vi "Client(UtilityMode).vi"() -> ()   [LabVIEW 2013, in "OPC UA Demo.lvlib"]
doc: "Demonstrates the use of the <B>OPC UA Client VIs</B> to programmatically create an OPC UA client and connects the OPC UA client to an OPC UA server."
uses:
  OPC UA Demo.lvlib
  <vilib>/OPCUA/client/Write Int32.vi
  <vilib>/OPCUA/NI OPC UA Client.lvlib
  OPCUA(Utility)/Client/OCPUA Client(UtilityMode).lvlib
panel:
  in  "Device.Node.Set Point":i32=1000
  out "error out":errorcluster
  out "Waveform Chart":i32(graph)
  in  "stop":bool
  # "Overview: Demonstrates the use of the OPC UA Client VIs to programmatically create an OPC UA client and connects the OPC UA client to an OPC UA server.\nRequirements: \n1. LabVIEW Datalogging and Supervisory Control Module or LabVIEW Real-Time Module\n2. (Real-Time Module) RT target\nInstructions:\nRun the VI."
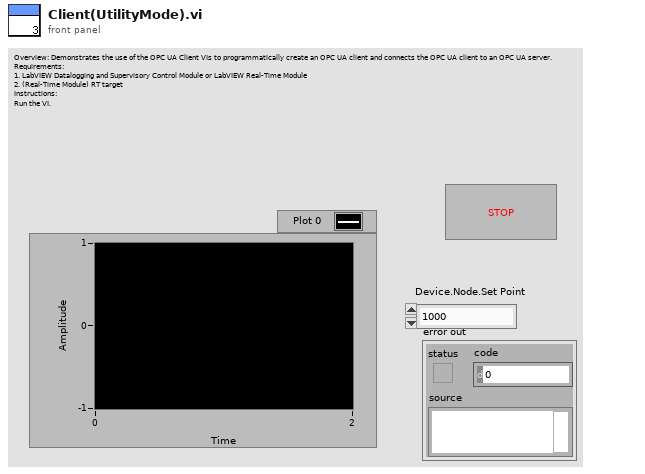
[diagram p1: front panel]
types:
  T1 = cluster{"Item URL":string, "Item Value":variant, "Timestamp":timestamp, "DataType":u32, "status code":u32}[]
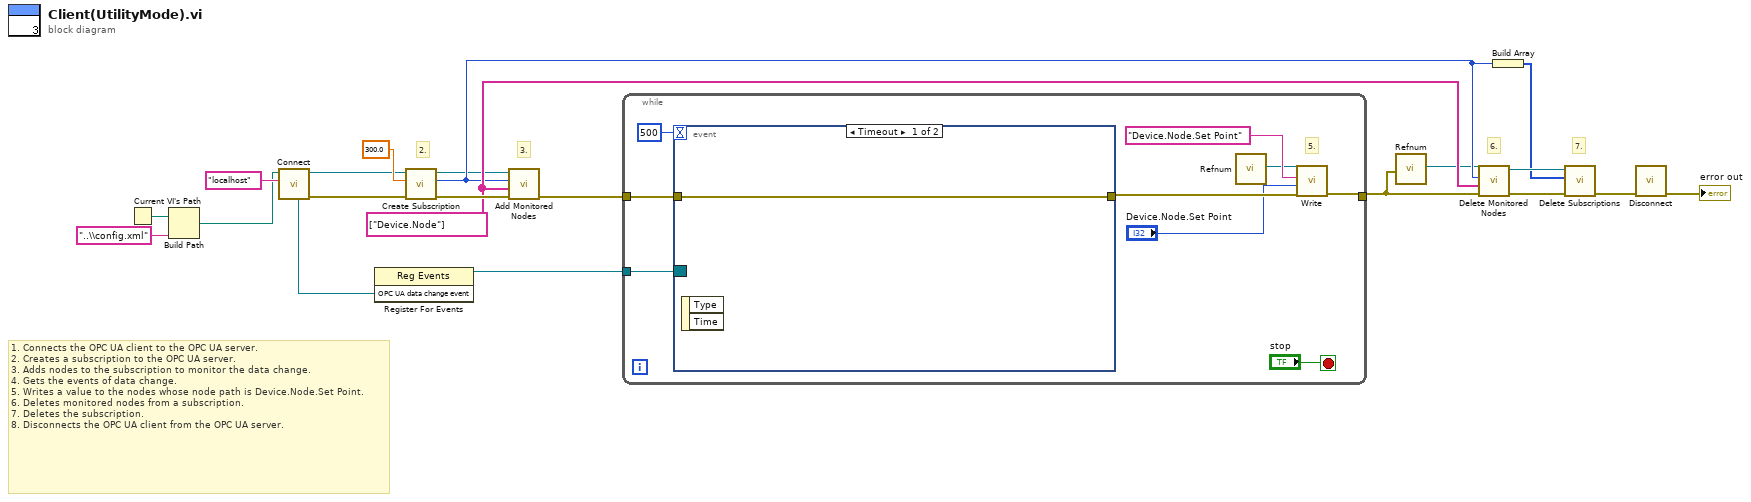
[diagram p0: block diagram]
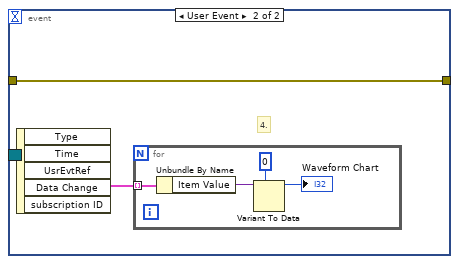
[diagram p2: hidden frame]
diagram:
  w15 = string[] ["Device.Node"] ("array of node path")
  # "7."
  # "1. Connects the OPC UA client to the OPC UA server. \n2. Creates a subscription to the OPC UA server.\n3. Adds nodes to the subscription to monitor the data change.\n4. Gets the events of data change.\n5. Writes a value to the nodes whose node path is Device.Node.Set Point. \n6. Deletes monitored nodes from a subscription.\n7. Deletes the subscription.\n8. Disconnects the OPC UA client from the OPC UA server."
  # "6."
  # "3."
  # "2."
  n1 = Current VI's Path() -> (path=w3:path)
  n2 = Build Path(base path=w3, name or relative path="..\\config.xml") -> (appended path=w1:path)
  n3 = call "Connect.vi"("Server IP"="localhost", "XML config File Path"=w1) -> ("error out"=w10:errorcluster, "OPC UA client refnum out"=w7:refnum<k21>, "OPC UA data change event"=w9:refnum<user-event>)  [unwired: 7 in]
  n4 = register-events(w9) -> (reference out=w20:refnum<event-registration>)  [unwired: 2 in, 1 out]
  n5 = call <vilib>:"Create Subscription.vi"("error in (no error)"=w10, "update rate (1000 ms)"=300.0, "OPC UA client refnum in"=w7) -> ("error out"=w21:errorcluster, "subscription ID out"=w14:u32, "OPC UA client refnum out"=w8:refnum<k21>)  [unwired: 6 in]
  n6 = call <vilib>:"Add Monitored Nodes.vi"("error in (no error)"=w21, "array of node path"=w15, "subscription ID in"=w14, "OPC UA client refnum in"=w8) -> ("error out"=w19:errorcluster)  [unwired: 5 in, 2 out]
  n7 = while {
    tunnel: w20 -> [w30]
    tunnel: w19 -> [w28]
    tunnel: [w26] -> w5
    stop <- "stop" stop-if-true
    # "5."
    n8 = event shown="[0] Timeout" {
      selector: w30 -> [_ _]
      dyn-events: _ -> [_ _]
      timeout: 500 -> [_ _]
      tunnel: w28 -> [w31 w33]
      tunnel: [w31 w33] -> w27
      event Timeout {
        n9 = event-data() -> ()  [unwired: 1 in, 2 out]
      }
      event User Event {
        # "4."
        n10 = event-data() -> ("Data Change"=w32:T1)  [unwired: 1 in, 4 out]
        n11 = for {
          tunnel: w32 -> [w37] mode=indexing
          n12 = Unbundle By Name(w37) -> ("Item Value"=w36:variant)
          n13 = Variant To Data(type=0, Variant=w36) -> (data=→"Waveform Chart":i32)  [unwired: 1 in, 1 out]
        }
      }
    }
    n14 = call "Refnum.vi"() -> ("OPC UA client refnum out"=w22:refnum<k21>)  [unwired: 18 in, 1 out]
    n15 = call-poly <vilib>:"Write.vi"("error in (no error)"=w27, "value"="Device.Node.Set Point", "node path"="Device.Node.Set Point", "OPC UA client refnum in"=w22) -> ("error out"=w26:errorcluster)  [unwired: 5 in, 2 out]
  }
  n16 = call "Refnum.vi"("error in (no error)"=w5) -> ("OPC UA client refnum out"=w6:refnum<k21>)  [unwired: 17 in, 1 out]
  n17 = call <vilib>:"Delete Monitored Nodes.vi"("error in (no error)"=w5, "array of node path"=w15, "subscription ID in"=w14, "OPC UA client refnum in"=w6) -> ("error out"=w17:errorcluster, "OPC UA client refnum out"=w18:refnum<k21>)  [unwired: 4 in, 2 out]
  n18 = Build Array(w14) -> (w13:u32[])
  n19 = call <vilib>:"Delete Subscriptions.vi"("error in (no error)"=w17, "array of subscription ID"=w13, "OPC UA client refnum in"=w18) -> ("error out"=w11:errorcluster)  [unwired: 6 in, 2 out]
  n20 = call "Disconnect.vi"("error in (no error)"=w11) -> ("error out"=→"error out":errorcluster)  [unwired: 10 in]
